vi "Combine Transliteration Maps.vi"(1 "new map":u8[](array[numeric]), 2 "map in":u8[](array[numeric])) -> (0 "map out":u8[](array[numeric]))   [LabVIEW 2009, in "Tools_String.lvlib"]
uses:
  Tools_String.lvlib
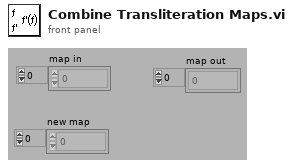
[diagram p1: front panel]
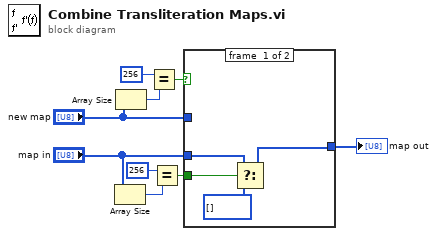
[diagram p0: block diagram]
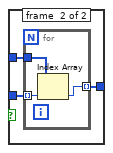
[diagram p3: hidden frame]
diagram:
  n1 = Array Size(array="map in") -> (size(s)=w4:i32)
  n2 = Array Size(array="new map") -> (size(s)=w8:i32)
  n3 = Equal?(x=256, y=w8) -> (x = y?=w6:bool)
  n4 = Equal?(x=256, y=w4) -> (x = y?=w2:bool)
  n5 = case shown="False" w6 {
    tunnel: "new map" -> [_ w17]
    tunnel: "map in" -> [w12 w15]
    tunnel: w2 -> [w13 w14]
    tunnel: [w11 w16] -> w1
    frame #0 {
      n6 = Select(t=w12, s=w13, f=u8[] []) -> (s? t:f=w11:u8[])
    }
    frame #1 {
      n7 = case shown="False" w14 {
        tunnel: w15 -> [_ w21]
        tunnel: [w18 w20] -> w16
        tunnel: w17 -> [w18 w19]
        frame #0 {
        }
        frame #1 {
          n8 = for {
            tunnel: w21 -> [w24] mode=indexing
            tunnel: w19 -> [w23]
            tunnel: [w22] -> w20 mode=indexing
            n9 = Index Array(array=w23, index=w24) -> (element=w22:u8)
          }
        }
      }
    }
  }
  "map out" <- w1
